vi "delta_2st.vi"(9 "c":dbl, 10 "b":dbl, 11 "a":dbl) -> (3 "Delta drugiego stopnia":dbl)   [LabVIEW 2020]
doc: "liczenie delty"
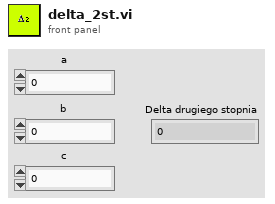
[diagram p1: front panel]
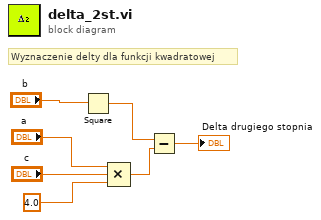
[diagram p0: block diagram]
diagram:
  # "Wyznaczenie delty dla funkcji kwadratowej"
  n1 = Square(x="b") -> (x^2=w4:dbl)
  n2 = Compound Arithmetic op=MULTIPLY("a", "c", 4.0 ("value")) -> (w3:dbl)
  n3 = Subtract(x=w4, y=w3) -> (x-y=→"Delta drugiego stopnia":dbl)
